vi "MI Cryostation 1.4 LV v10.vi"(4 "Checking interval (s)":u32, 5 "Precision":dbl=0.1 format="%#_13g", 6 "Timeout (s)":i32=600, 7 "Trials":i32=3, 8 "error in (no error)":errorcluster, 9 "Temperature Set Point":dbl=4.2 min=2.0 max=350.0 step=1.0 format="%.2f", 10 "Command":string="03GPT", 11 "Address":string="10.0.0.3") -> (0 "error out":errorcluster, 1 "Current temp":dbl)   [LabVIEW 2016, in "MyMontana.lvlib"]
doc: "Displays data sent via TCP from Data Server.vi. Once a TCP connection is open, the VI reads 4 bytes to determine the amount of data being sent. It then reads and charts that many bytes. If an error occurs or the stop button is pressed, it sends a \"Q\" to the Data Sender to notify it to quit.\n\n<B>Note:</B> Requires the Data Server.vi located in the same library as this VI."
uses:
  MyMontana.lvlib
panel:
  # "Input the IP address of the Cryostation PC"
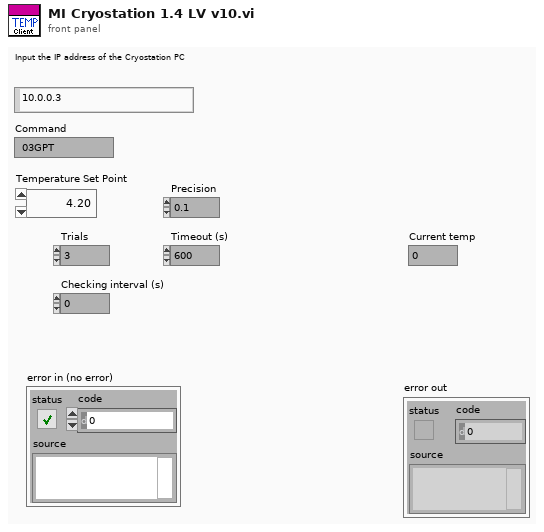
[diagram p1: front panel]
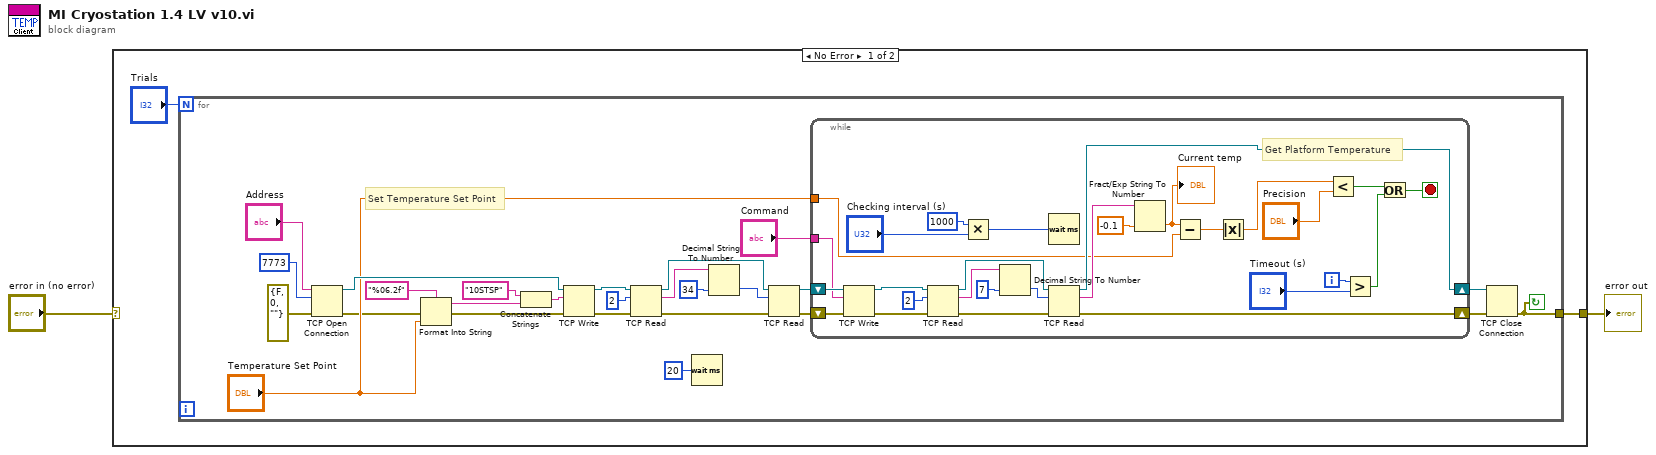
[diagram p0: block diagram]
diagram:
  n1 = case shown="No Error" "error in (no error)" {
    selector: "error in (no error)" -> [_ w59]
    tunnel: [w3 w59] -> w1
    frame No Error {
      n2 = for {
        N: "Trials" -> [_]
        tunnel: [w6] -> w3
        stop <- w6 continue-if-true
        # "Set Temperature Set Point"
        n3 = TCP Open Connection(address="Address", remote port or service name=u16 7773, error in (no error)=errorcluster {"status"=FALSE, "code"=0, "source"=""}) -> (connection ID=w29:refnum<k5>, error out=w11:errorcluster)  [unwired: 2 in]
        n4 = Format Into String(format string="%06.2f", error in=w11, "Temperature Set Point") -> (resulting string=w23:string, error out=w10:errorcluster)  [unwired: 1 in]
        n5 = Concatenate Strings("10STSP", w23) -> (w22:string)
        n6 = TCP Write(connection ID=w29, data in=w22, error in (no error)=w10) -> (connection ID out=w21:refnum<k5>, error out=w16:errorcluster)  [unwired: 1 in, 1 out]
        n7 = TCP Read(connection ID=w21, bytes to read=2 ("timeout ms (25000)"), error in (no error)=w16) -> (connection ID out=w19:refnum<k5>, data out=w18:string, error out=w15:errorcluster)  [unwired: 2 in]
        n8 = Wait (ms)(milliseconds to wait=u32 20) -> ()  [unwired: 1 out]
        n9 = Decimal String To Number(string=w18, default (0L)=34 ("default (0 I32)")) -> (number=w17:i32)  [unwired: 1 in, 1 out]
        n10 = TCP Read(connection ID=w19, bytes to read=w17, error in (no error)=w15) -> (connection ID out=w13:refnum<k5>, error out=w9:errorcluster)  [unwired: 2 in, 1 out]
        n11 = while {
          shift-right: [w47] -> w27
          shift-left: w13 -> [w48]
          tunnel: "Temperature Set Point" -> [w45]
          tunnel: "Command" -> [w37]
          shift-right: [w34] -> w8
          shift-left: w9 -> [w35]
          i -> [w41]
          stop <- w36 stop-if-true
          # "Get Platform Temperature"
          n12 = TCP Write(connection ID=w48, data in=w37, error in (no error)=w35) -> (connection ID out=w58:refnum<k5>, error out=w52:errorcluster)  [unwired: 1 in, 1 out]
          n13 = TCP Read(connection ID=w58, bytes to read=2, error in (no error)=w52) -> (connection ID out=w55:refnum<k5>, data out=w56:string, error out=w51:errorcluster)  [unwired: 2 in]
          n14 = Multiply(x=u32 1000, y="Checking interval (s)") -> (x*y=w31:u32)
          n15 = Decimal String To Number(string=w56, default (0L)=7 ("default (0 I32)")) -> (number=w54:i32)  [unwired: 1 in, 1 out]
          n16 = Wait (ms)(milliseconds to wait=w31) -> ()  [unwired: 1 out]
          n17 = TCP Read(connection ID=w55, bytes to read=w54, error in (no error)=w51) -> (connection ID out=w47:refnum<k5>, data out=w53:string, error out=w34:errorcluster)  [unwired: 2 in]
          n18 = Fract/Exp String To Number(string=w53, default (0 dbl)=-0.1 ("default (0 DBL)")) -> (number=w46:dbl)  [unwired: 2 in, 1 out]
          "Current temp" <- w46
          n19 = Subtract(x=w46, y=w45) -> (x-y=w44:dbl)
          n20 = Absolute Value(x=w44) -> (abs(x)=w43:dbl)
          n21 = Less?(x=w43, y="Precision") -> (x < y?=w38:bool)
          n22 = Greater?(x=w41, y="Timeout (s)") -> (0:w39:bool)
          n23 = Or(x=w38, y=w39) -> (x .or. y?=w36:bool)
        }
        n24 = TCP Close Connection(connection ID=w27, error in (no error)=w8) -> (error out=w6:errorcluster)  [unwired: 1 in, 1 out]
      }
    }
    frame Error {
    }
  }
  "error out" <- w1
